vi "Transmission Model.vi"(8 "Transmission Speed Out (rad/s)":sgl, 9 "Vehicle Speed (mph)":sgl, 10 "Engine Speed (rad/s)":sgl, 11 "Throttle (%)":sgl) -> (1 "Gear":sgl, 2 "Impeller Torque (N-m)":sgl, 3 "Transmission Torque Out (N-m)":sgl)   [LabVIEW 2016, in "NI-PCG Vehicle Model.lvlib"]
uses:
  NI-PCG Vehicle Model.lvlib
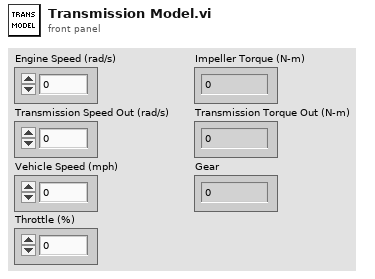
[diagram p1: front panel]
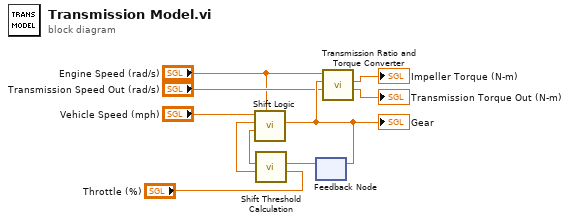
[diagram p0: block diagram]
diagram:
  n1 = feedback #1() -> (w10:sgl)  [unwired: 1 in]
  n2 = call "Shift Threshold Calculation.vi"("Throttle (%)"="Throttle (%)", "Gear"=w10) -> ("Up Threshold (mph)"=w9:sgl, "Down Threshold (mph)"=w8:sgl)  [unwired: 8 in]
  n3 = call "Shift Logic.vi"("Engine Speed (rad/s)"="Engine Speed (rad/s)", "Down Threshold"=w8, "Up Threshold"=w9, "Vehicle Speed (mph)"="Vehicle Speed (mph)") -> ("Gear"=w6:sgl)  [unwired: 7 in]
  "Gear" <- w6
  n4 = feedback-in #1(w6) -> ()
  n5 = call "Transmission Ratio and Torque Converter.vi"("Transmission Speed Out (rad/s)"="Transmission Speed Out (rad/s)", "Gear"=w6, "Impeller Speed (rad/s)"="Engine Speed (rad/s)") -> ("Transmission Torque Out (N-m)"=→"Transmission Torque Out (N-m)":sgl, "Impeller Torque (N-m)"=→"Impeller Torque (N-m)":sgl)  [unwired: 7 in]
